vi "Find Open Dir.vi"(8 "error in (no error)":errorcluster, 11 "dir in":refnum<class "dir.lvclass">) -> (0 "error out":errorcluster, 2 "open dir":refnum<class "dir.lvclass">, 3 "dir out":refnum<class "dir.lvclass">)   [LabVIEW 2023, in "d7.lvlib" / "dir.lvclass"]
uses:
  dir.lvclass
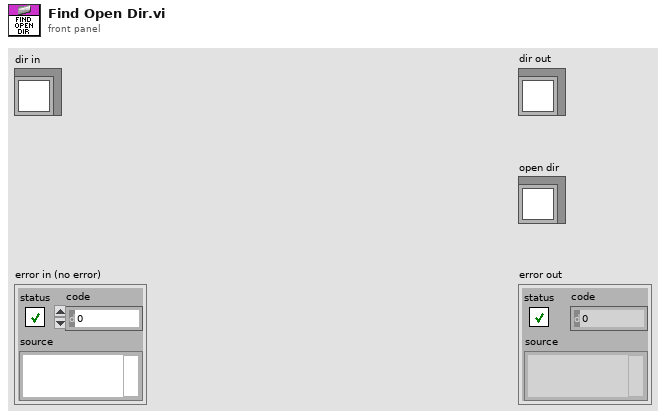
[diagram p1: front panel]
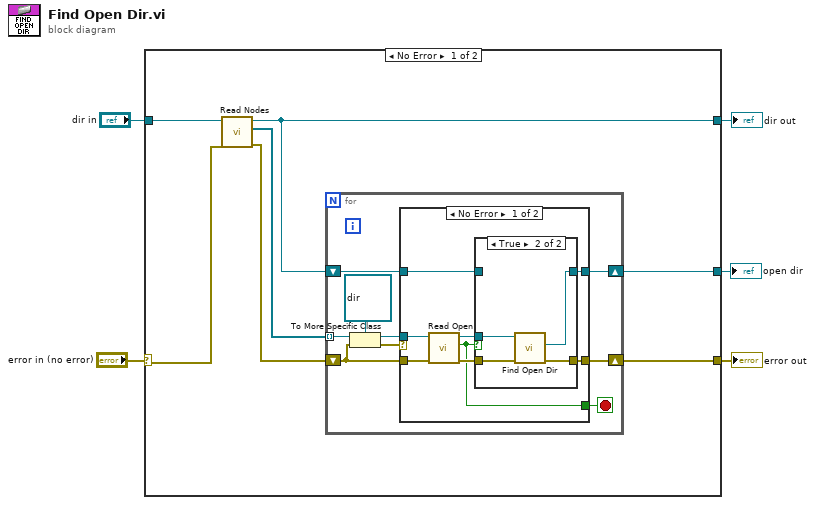
[diagram p0: block diagram]
diagram:
  n1 = case shown="No Error" "error in (no error)" {
    selector: "error in (no error)" -> [w10 w38]
    tunnel: "dir in" -> [w8 w39]
    tunnel: [w9 w39] -> w4
    tunnel: [w12 _] -> w2
    tunnel: [w11 w38] -> w1
    frame No Error {
      n2 = call-dynamic "Read Nodes.vi"("error in (no error)"=w10, "dir in"=w8) -> ("error out"=w7:errorcluster, "Nodes"=w6:refnum<class "INode.lvclass">[], "dir out"=w9:refnum<class "dir.lvclass">)  [unwired: 7 in]
      n3 = for {
        tunnel: w6 -> [w18] mode=indexing
        shift-right: [w15] -> w11
        shift-left: w7 -> [w16]
        shift-right: [w17] -> w12
        shift-left: w9 -> [w13]
        stop <- w14 stop-if-true
        n4 = To More Specific Class(target class=refnum<class "dir.lvclass"> refnum ("d7.lvlib:dir.lvclass"), reference=w18, error in=w16) -> (specific class reference=w20:refnum<class "dir.lvclass">, error out=w19:errorcluster)
        n5 = case shown="No Error" w19 {
          tunnel: w20 -> [w26 _]
          tunnel: w13 -> [w22 w37]
          tunnel: [w29 w37] -> w17
          tunnel: w16 -> [w24 w36]
          tunnel: [w28 w36] -> w15
          tunnel: [w23 _] -> w14
          frame No Error {
            n6 = call-dynamic "Read Open.vi"("error in (no error)"=w24, "dir in"=w26) -> ("error out"=w25:errorcluster, "Open"=w23:bool, "dir out"=w27:refnum<class "dir.lvclass">)  [unwired: 7 in]
            n7 = case shown="True" w23 {
              tunnel: [w31 w35] -> w29
              tunnel: [w30 w34] -> w28
              tunnel: w27 -> [_ w33]
              tunnel: w25 -> [w30 w32]
              tunnel: w22 -> [w31 _]
              frame False {
              }
              frame True {
                n8 = call "Find Open Dir.vi"("error in (no error)"=w32, "dir in"=w33) -> ("error out"=w34:errorcluster, "open dir"=w35:refnum<class "dir.lvclass">)  [unwired: 7 in, 1 out]
              }
            }
          }
          frame Error {
          }
        }
      }
    }
    frame Error {
    }
  }
  "error out" <- w1
  "open dir" <- w2
  "dir out" <- w4
